vi "ConfigUtilities - Add System Mapping.vi"(8 "error in (no error)":errorcluster, 9 "Channel Path Destination":string, 10 "Channel Path Source":string, 11 "Item Ref in":T1 format="%.0x") -> (0 "error out":errorcluster, 3 "Item Ref out":T1 format="%.0x")   [LabVIEW 2016, in "UDP-Custom-Device System Explorer.lvlib"]
uses:
  UDP-Custom-Device System Explorer.lvlib
  <vilib>/NI Veristand/Custom Device API/Custom Device Item Ref.ctl
  NationalInstruments.VeriStand.SystemDefinitionAPI
  <vilib>/NI VeriStand/Custom Device API/Custom Device API.lvlib
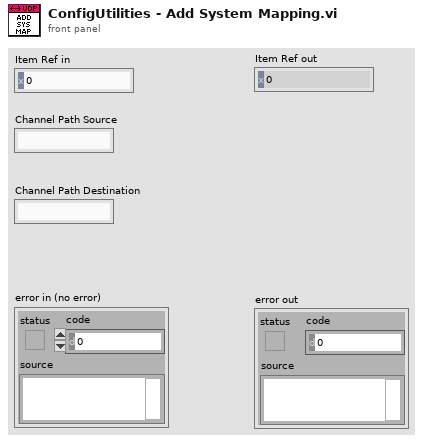
[diagram p1: front panel]
types:
  T1 = typedef "Custom Device API.lvlib/Custom Device Item Ref.ctl" = u64
  T2 = typedef "Custom Device API.lvlib/Custom Device Pointer.ctl" = refnum<k24>
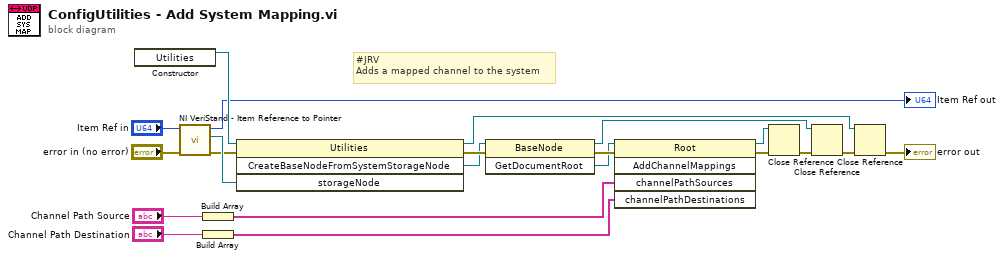
[diagram p0: block diagram]
diagram:
  # "#JRV\nAdds a mapped channel to the system"
  n1 = constructor class="Utilities"() -> (reference out=w10:refnum<k24>)  [unwired: 3 in, 2 out]
  n2 = call <vilib>:"NI VeriStand - Item Reference to Pointer.vi"("error in (no error)"="error in (no error)", "Item Ref in"="Item Ref in") -> ("error out"=w8:errorcluster, "Node Pointer"=w9:T2, "Item Ref out"=→"Item Ref out":T1)  [unwired: 6 in, 1 out]
  n3 = Build Array("Channel Path Source") -> (w3:string[])
  n4 = Build Array("Channel Path Destination") -> (w1:string[])
  n5 = invoke class="Utilities" method="CreateBaseNodeFromSystemStorageNode"(reference=w10, error in=w8, "storageNode"=w9) -> (reference out=w20:refnum<k24>, error out=w13:errorcluster, "CreateBaseNodeFromSystemStorageNode"=w11:refnum<k24>)  [unwired: 1 in, 1 out]
  n6 = invoke class="BaseNode" method="GetDocumentRoot"(reference=w11, error in=w13) -> (reference out=w18:refnum<k24>, error out=w14:errorcluster, "GetDocumentRoot"=w12:refnum<k24>)  [unwired: 1 in]
  n7 = invoke class="Root" method="AddChannelMappings"(reference=w12, error in=w14, "channelPathSources"=w3, "channelPathDestinations"=w1) -> (reference out=w16:refnum<k24>, error out=w15:errorcluster)  [unwired: 1 in, 3 out]
  n8 = Close Reference(reference=w16, error in (no error)=w15) -> (error out=w17:errorcluster)
  n9 = Close Reference(reference=w18, error in (no error)=w17) -> (error out=w19:errorcluster)
  n10 = Close Reference(reference=w20, error in (no error)=w19) -> (error out=→"error out":errorcluster)
